vi "Set Shutter Closing Time.vi"(8 "error in (no error)":errorcluster, 11 "CCDCamera in":refnum<class "CCDCamera.lvclass">) -> (0 "error out":errorcluster, 3 "CCDCamera out":refnum<class "CCDCamera.lvclass">)   [LabVIEW 2018]
uses:
  Simulated_CCD_Camera/Simulated_CCD_Camera.lvclass
  Interface/Interface.lvclass
  CCDCamera.lvclass
  C:/Users/observer/Desktop/SPARC4_ACS/SPARC4_ACS/Simulated_CCD_Camera/Simulated_CCD_Camera.lvclass
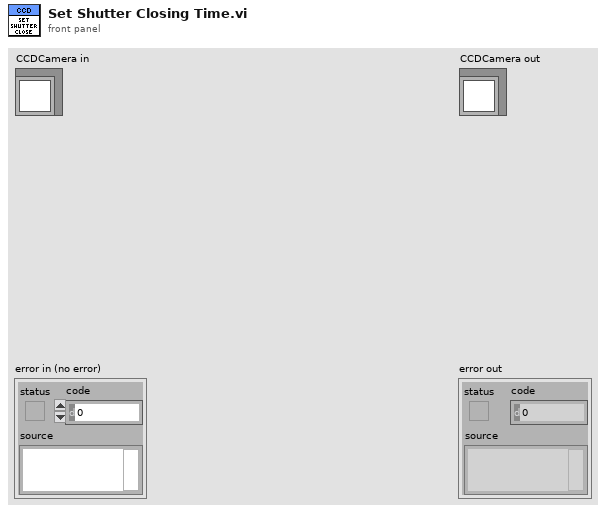
[diagram p1: front panel]
types:
  T1 = cluster{"PREAMP":u16, "READOUT_RATE":u16, "EM_GAIN":u16, "VBIN":u16, "INITIAL_LINE":u16, "INITIAL_COLUMN":u16, "FINAL_LINE":u16, "FINAL_COLUMN":u16, "TRIGGER_MODE":u16, "HBIN":u16, "SHUTTER_TTL":u16, "SHUTTER_MODE":u16, "SHUTTER_OPENING_TIME":u16, "SHUTTER_CLOSING_TIME":u16, "VERTICAL_SHIFT_SPEED":u16, "READ_MODE":u16, "FRAME_TRANSFER":bool, "VERTICAL_CLOCK_VOLTAGE":u16, "ACQUISITION_MODE":u16, "AD_CHANNEL":u16, "EM_MODE":u16}
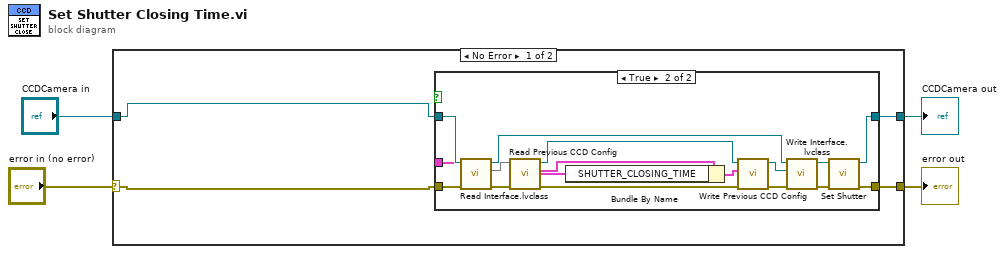
[diagram p0: block diagram]
diagram:
  n1 = case shown="No Error" "error in (no error)" {
    selector: "error in (no error)" -> [w5 w28]
    tunnel: [w7 w28] -> w1
    tunnel: [w6 w27] -> w2
    tunnel: "CCDCamera in" -> [w8 w27]
    frame No Error {
      n2 = case shown="True" {
        selector: _ -> [_ _]
        tunnel: w8 -> [w10 w13]
        tunnel: [w9 w15] -> w7
        tunnel: [w10 w14] -> w6
        tunnel: w5 -> [w9 w12]
        tunnel: _ -> [_ w11]
        frame False {
        }
        frame True {
          n3 = call "Read Interface.lvclass.vi"("error in (no error)"=w12, "Simulated_CCD_Camera in"=w13) -> ("error out"=w18:errorcluster, 2:w22, "Simulated_CCD_Camera out"=w20:refnum<class "CCDCamera.lvclass">)  [unwired: 7 in]
          n4 = call "Read Previous CCD Config.vi"("error in (no error)"=w18, "Interface in"=w22) -> ("error out"=w24:errorcluster, "CCD Config"=w26:T1, "Interface out"=w23:refnum<class "Interface.lvclass">)  [unwired: 7 in]
          n5 = Bundle By Name(cluster=w26, "SHUTTER_CLOSING_TIME"=w11) -> (w25:T1)
          n6 = call "Write Previous CCD Config.vi"("error in (no error)"=w24, "CCD Config"=w25, "Interface in"=w23) -> ("error out"=w19:errorcluster, "Interface out"=w21:refnum<class "Interface.lvclass">)  [unwired: 7 in]
          n7 = call "Write Interface.lvclass.vi"("error in (no error)"=w19, "Interface.lvclass"=w21, "Simulated_CCD_Camera in"=w20) -> ("error out"=w16:errorcluster, "Simulated_CCD_Camera out"=w17:refnum<class "CCDCamera.lvclass">)  [unwired: 7 in]
          n8 = call-dynamic "Set Shutter.vi"("error in (no error)"=w16, "CCDCamera in"=w17) -> ("error out"=w15:errorcluster, "CCDCamera out"=w14:refnum<class "CCDCamera.lvclass">)  [unwired: 8 in]
        }
      }
    }
    frame Error {
    }
  }
  "error out" <- w1
  "CCDCamera out" <- w2
